vi "timer_fgv.vi"(9 "Operation":T1, 10 "TImer":dbl) -> (2 "TIme passed?":bool)   [LabVIEW 2022 SP3]
uses:
  ctl_timer_fgv_states_enum.ctl
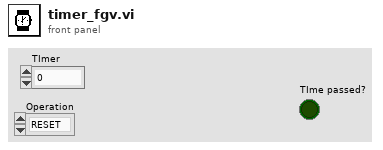
[diagram p1: front panel]
types:
  T1 = typedef "ctl_timer_fgv_states_enum.ctl" = enum16{"RESET", "GET"}
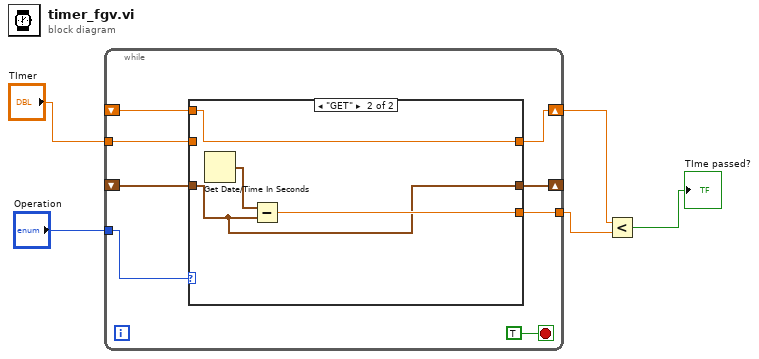
[diagram p0: block diagram]
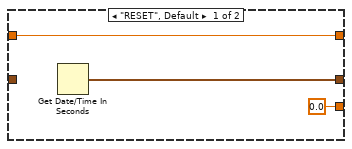
[diagram p2: hidden frame]
diagram:
  n1 = while {
    tunnel: "Operation" -> [w11]
    tunnel: "TImer" -> [w12]
    shift-right: [w10] -> _
    shift-left: _ -> [w9]
    shift-right: [w8] -> w2
    shift-left: _ -> [w7]
    tunnel: [w6] -> w3
    stop <- TRUE stop-if-true
    n2 = case shown="\"GET\"" w11 {
      tunnel: w12 -> [w15 _]
      tunnel: [w16 w17] -> w10
      tunnel: w9 -> [_ w17]
      tunnel: [w15 w18] -> w8
      tunnel: w7 -> [_ w18]
      tunnel: [0.0 w19] -> w6
      frame "RESET", Default {
        n3 = Get Date/Time In Seconds() -> (seconds since 1Jan1904=w16:timestamp)
      }
      frame "GET" {
        n4 = Get Date/Time In Seconds() -> (seconds since 1Jan1904=w20:timestamp)
        n5 = Subtract(x=w20, y=w17) -> (x-y=w19:dbl)
      }
    }
  }
  n6 = Less?(x=w2, y=w3) -> (x < y?=→"TIme passed?":bool)
